vi "ifr2025 PM.vi"(4 "State (Off)":bool, 5 "Source (INT)":i16(ring) items=["INT", "EXT AC", "EXT ALC", "EXT DC"], 6 "Waveform (Sine)":i16(ring) items=["Sine", "Triangle", "Square"], 7 "Mod Rate (400)":dbl=400.0, 8 "error in (no error)":errorcluster {"code" format="%.0x"}, 9 "Deviation (0.00)":dbl, 10 "Channel (PM1)":bool=TRUE, 11 "instrument handle":refnum<visa-resource-name>) -> (0 "error out":errorcluster {"code" format="%.0x"}, 3 "instrument handle out":refnum<visa-resource-name>)   [LabVIEW 2009]
doc: "Allows either of the two PM modulation sources to be configured."
uses:
  Ifr2025_32.dll
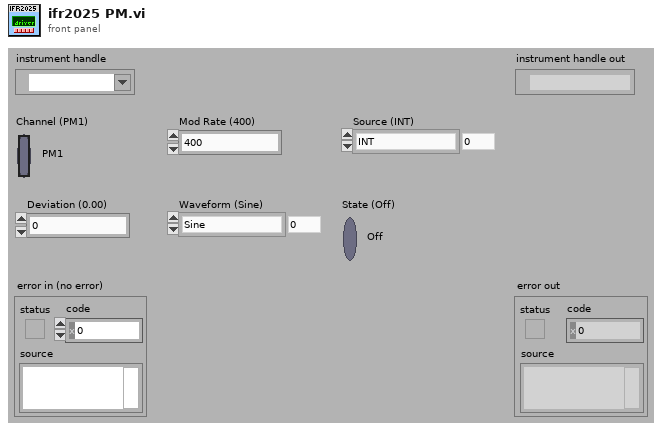
[diagram p1: front panel]
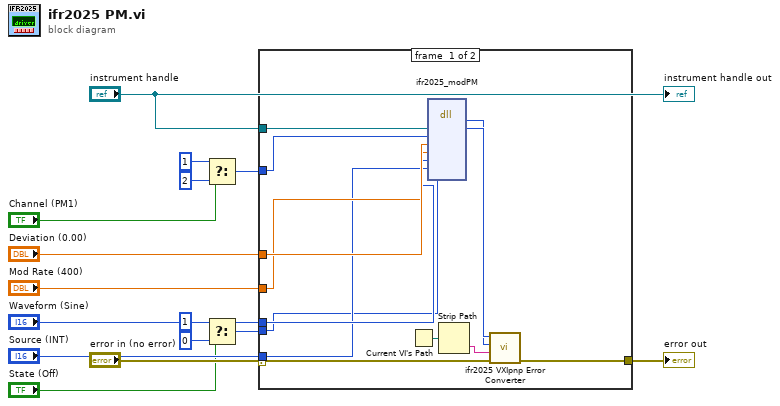
[diagram p0: block diagram]
diagram:
  n1 = Select(t=i16 1, s="Channel (PM1)", f=i16 2) -> (s? t:f=w9:i16)
  n2 = Select(t=u16 1, s="State (Off)", f=u16 0) -> (s? t:f=w1:u16)
  n3 = case shown="No Error" "error in (no error)" {
    selector: "error in (no error)" -> [w23 w29]
    tunnel: [w22 w29] -> w15
    tunnel: "instrument handle" -> [w27 _]
    tunnel: w9 -> [w21 _]
    tunnel: "Deviation (0.00)" -> [w20 _]
    tunnel: "Mod Rate (400)" -> [w19 _]
    tunnel: "Waveform (Sine)" -> [w18 _]
    tunnel: "Source (INT)" -> [w17 _]
    tunnel: w1 -> [w16 _]
    frame #0 {
      n4 = Current VI's Path() -> (path=w28:path)
      n5 = dll-call lib="P:/inst/Marconi 2024 Signal Generator/source/labview/ifr2025/ifr2025/ifr2025_*.*" fn="ifr2025_modPM"("vi"=w27, "Channel"=w21, "Deviation"=w20, "Mod Rate"=w19, "Waveform"=w18, "Source"=w17, "State"=w16) -> (w25:i32, "vi"=w26:u32)  [unwired: 9 in, 2 out]
      n6 = Strip Path(path=w28) -> (name=w24:string)  [unwired: 1 out]
      n7 = call "ifr2025 VXIpnp Error Converter.vi"("error in (no error)"=w23, "name of VI (\"\")"=w24, "CVI error code (0)"=w25, "instrument handle"=w26) -> ("error out"=w22:errorcluster)  [unwired: 7 out]
    }
    frame #1 {
    }
  }
  "error out" <- w15
  "instrument handle out" <- "instrument handle"
